vi "Main.vi"() -> ()   [LabVIEW 2016]
doc: "This template is for the Queued Message Handler design pattern.\n\nThe Event Handling Loop generates messages based on user interface actions.\n\nThe Message Handling Loop processes messages generated by the Event Handling Loop, or by other messages. The messages are string values, so new messages can be added easily to the Message Cases case structure in the Message Handling Loop. Each message cluster can also provide an optional value for Message Data, which is a variant that can be converted to whatever message-specific data is required."
uses:
  <vilib>/Utility/error.llb/Error Cluster From Error Code.vi
  <vilib>/ErrorRing/Error Ring.xnode
  3.SubVI/Message Queue/Message Queue.lvlib
panel:
  in  "Tab Control":enum32{"Page 1", "Page 2"}(tab)
  out "Display":string
  in  "Cancel Button":bool
  in  "原點復歸1":bool
  in  "生產結束":bool
  in  "Recipe":bool
  in  "Setting":bool
  in  "System":bool
  in  "停止":bool
  in  "啟動":bool
  out "X":dbl
  out "Y":dbl
  out "ON/OFF":bool
  in  "Pause":bool
  out "Speed":dbl
  in  "入料":bool
  in  "入料 2":bool
  out "Speed 2":dbl
  out "Y 2":dbl
  out "X 2":dbl
  out "ON/OFF 2":bool
  out "Display  2":string
  in  "原點復歸2":bool
  in  "Pause 2":bool
  in  "Cancel Button 2":bool
  in  "復歸":bool
  in  "SVON":bool
  in  "U":bool
  in  "D":bool
  in  "L":bool
  in  "R":bool
  in  "Step Ring 2":u16(ring) items=["0.001 mm", "0.01 mm", "0.1 mm", "1 mm"]
  in  "Jog_Speed":i32=10000
  # "工具列"
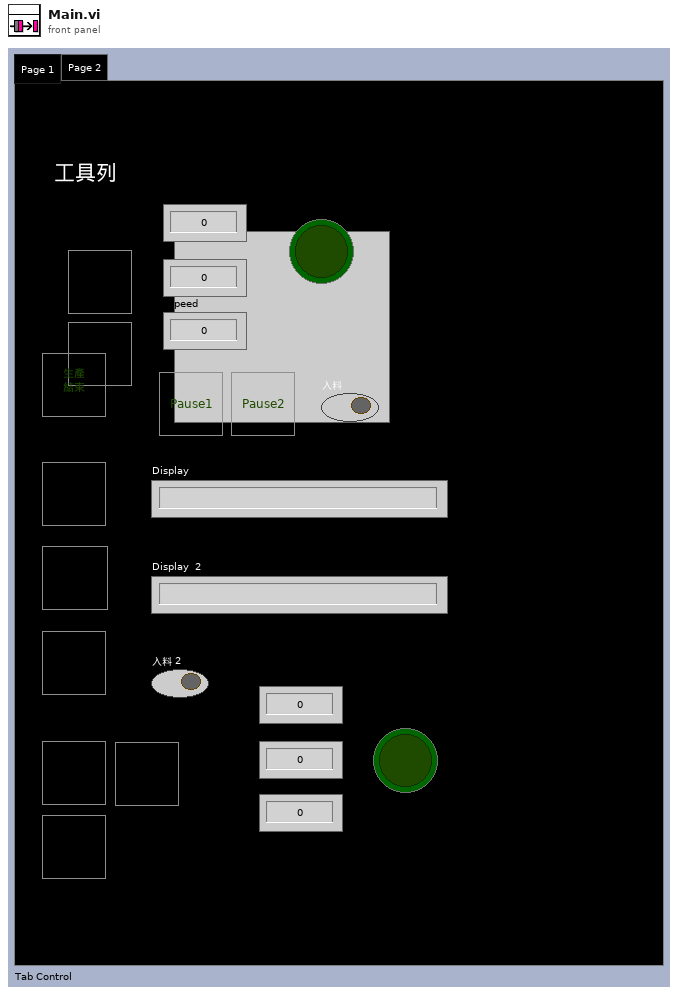
[diagram p1: front panel]
types:
  T1 = enum16{"Open", "Enqueue", "InsertQueue", "Release Queue", "Close"}
  T2 = enum16{"Open", "Move", "Check done", "E.Stop", "Get posion", "Home", "Serv ON/OFF", "Reset Error", "Set Param", "Close"}
  T3 = cluster{"X":dbl, "Y":dbl, "Speed":dbl, "Message":string}[]
  T4 = cluster{"X":dbl, "Y":dbl, "Speed":dbl, "Message":string}
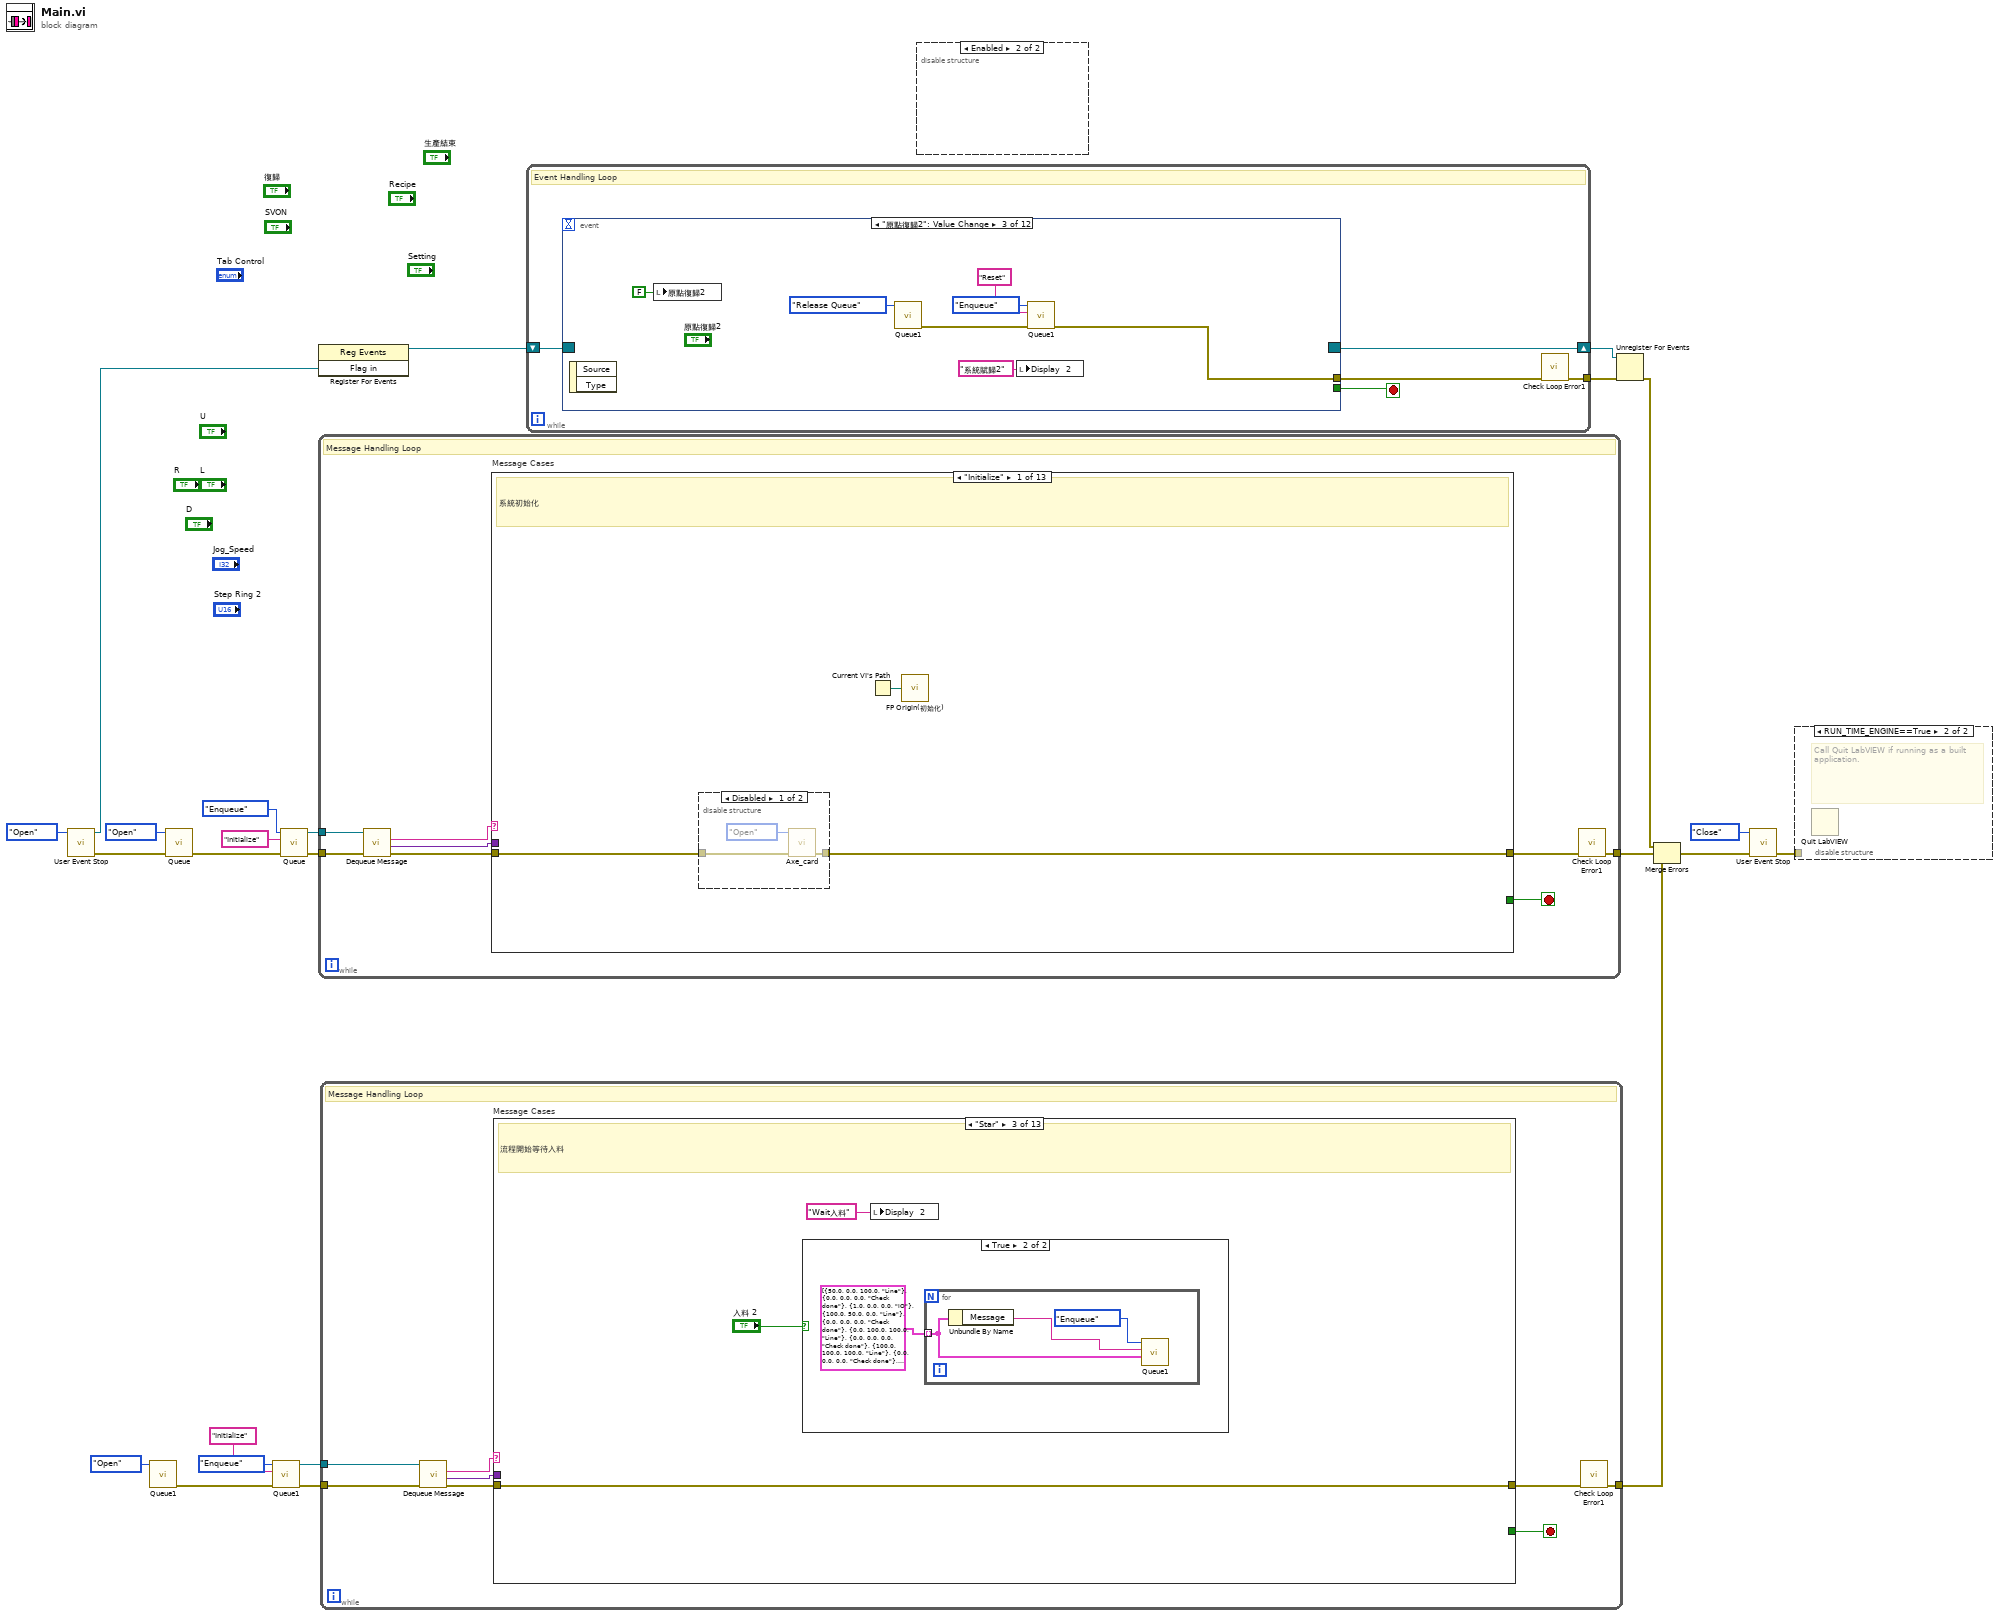
[diagram p0: block diagram]
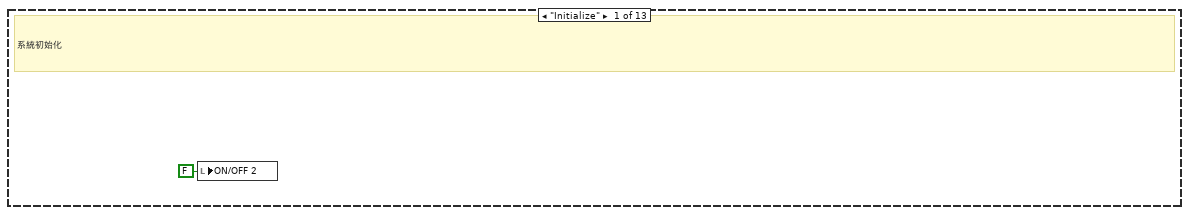
[diagram p2: hidden frame]
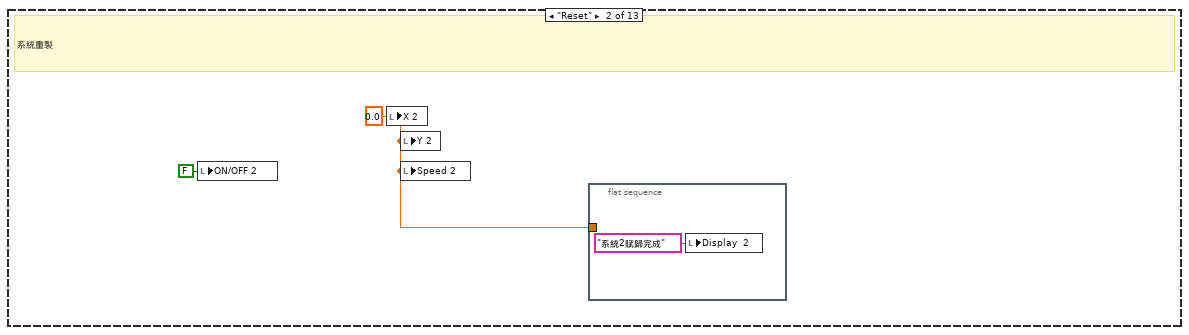
[diagram p3: hidden frame]
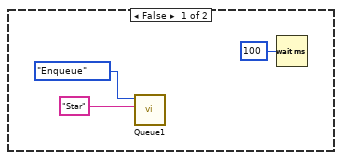
[diagram p4: hidden frame]
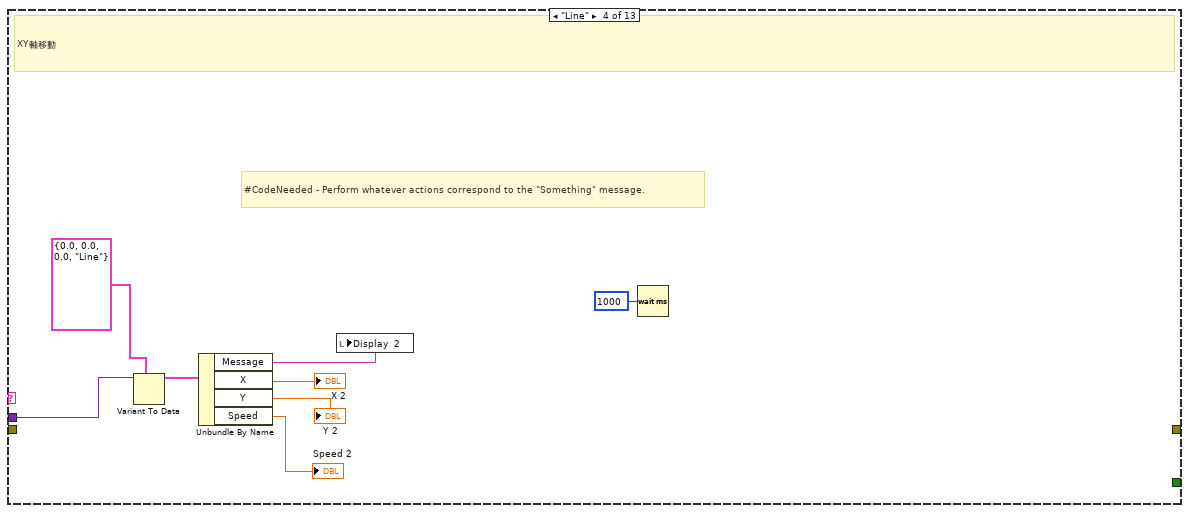
[diagram p5: hidden frame]
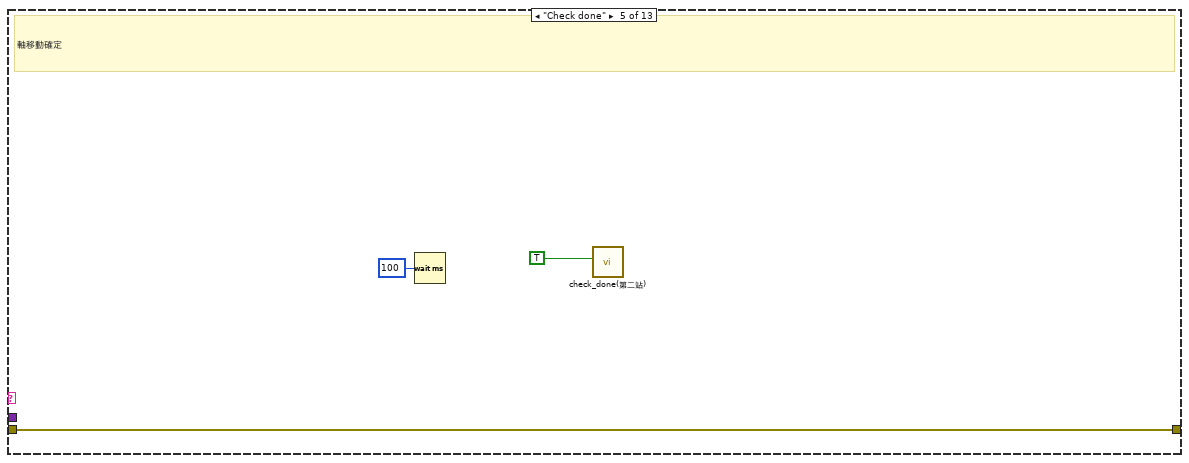
[diagram p6: hidden frame]
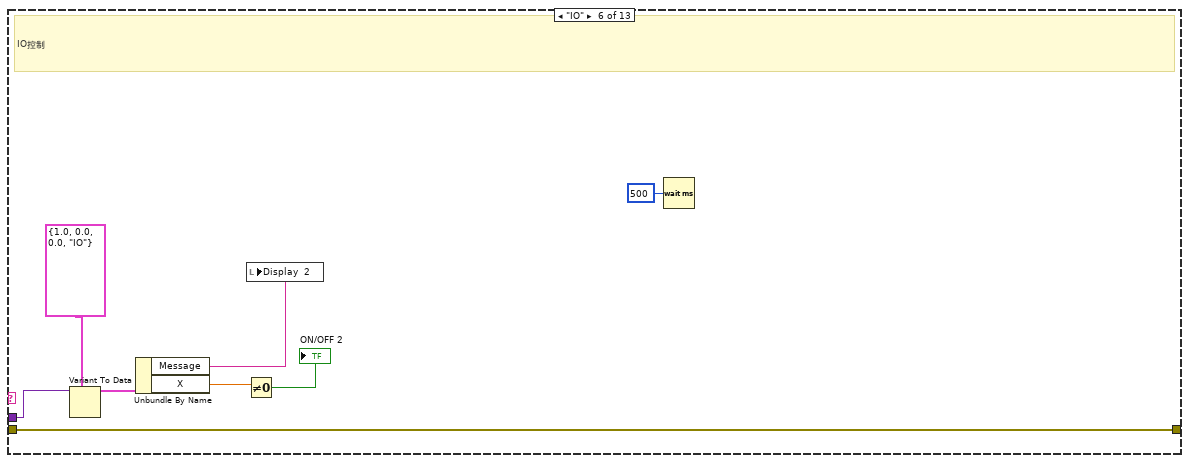
[diagram p7: hidden frame]
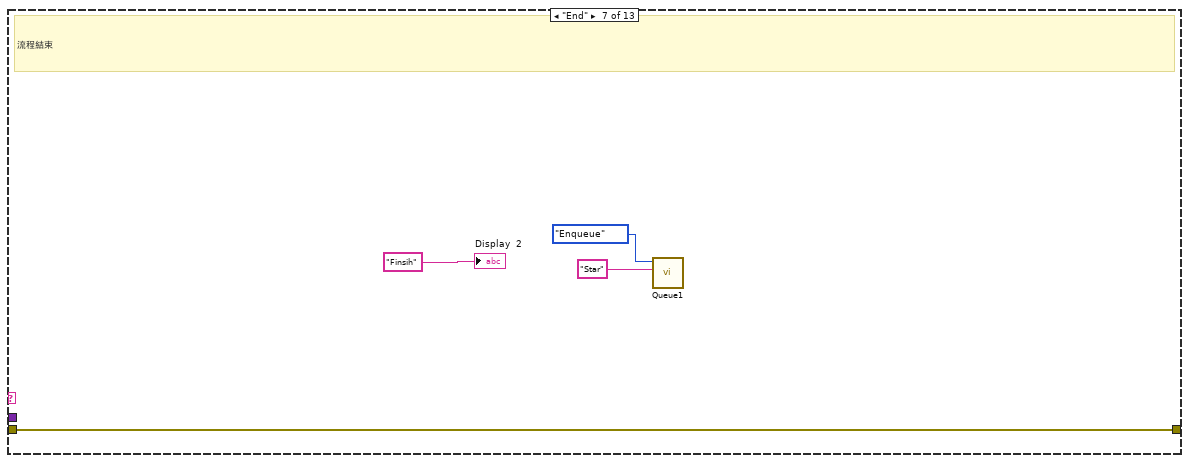
[diagram p8: hidden frame]
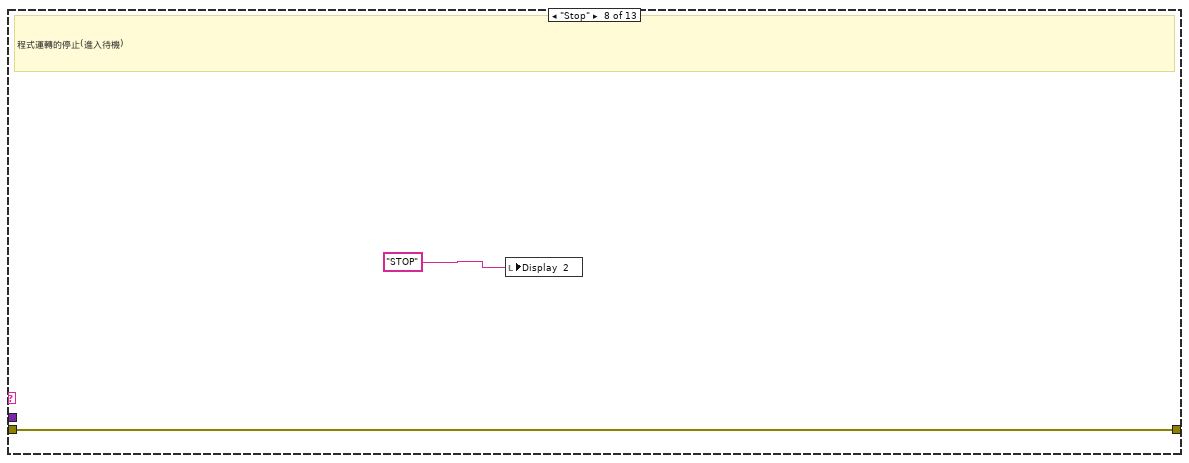
[diagram p9: hidden frame]
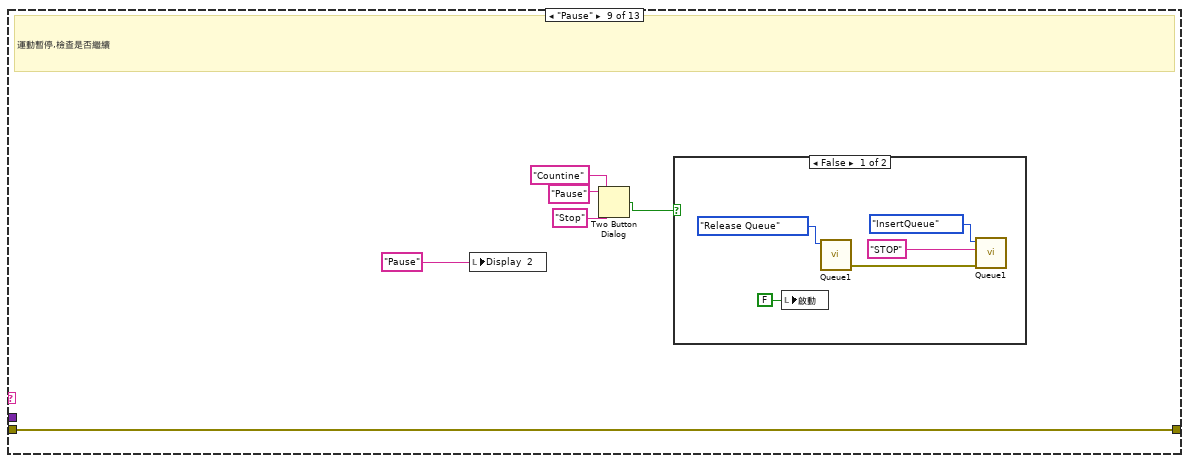
[diagram p10: hidden frame]
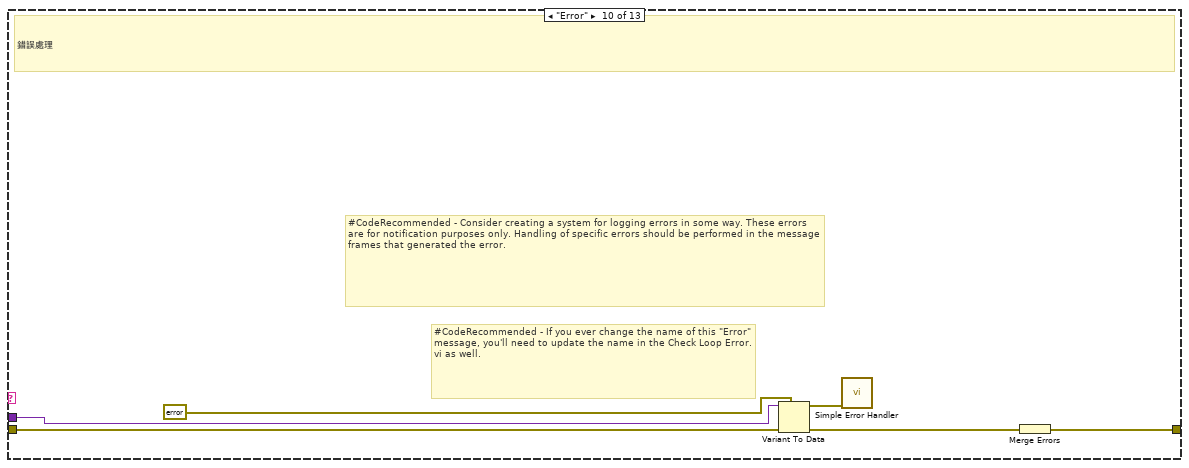
[diagram p12: hidden frame]
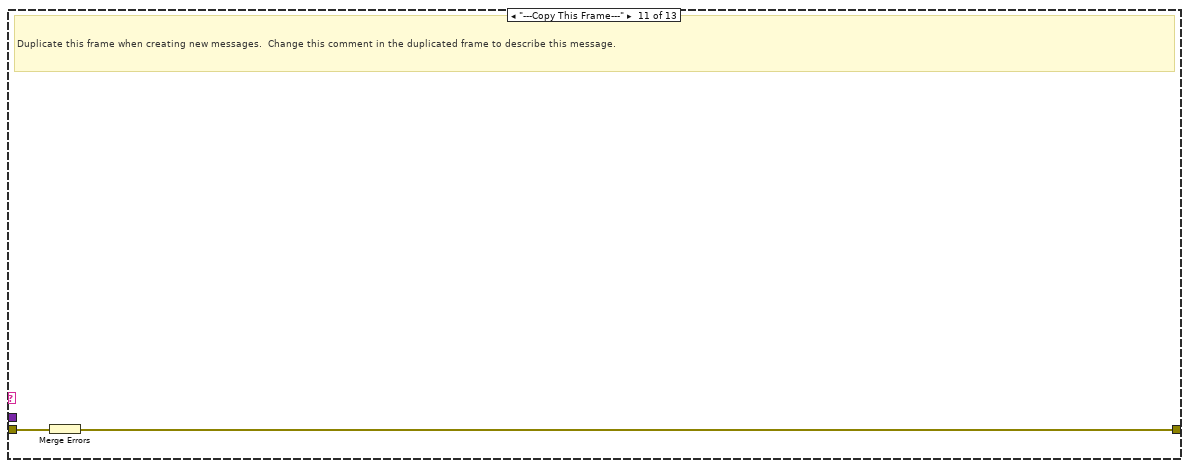
[diagram p13: hidden frame]
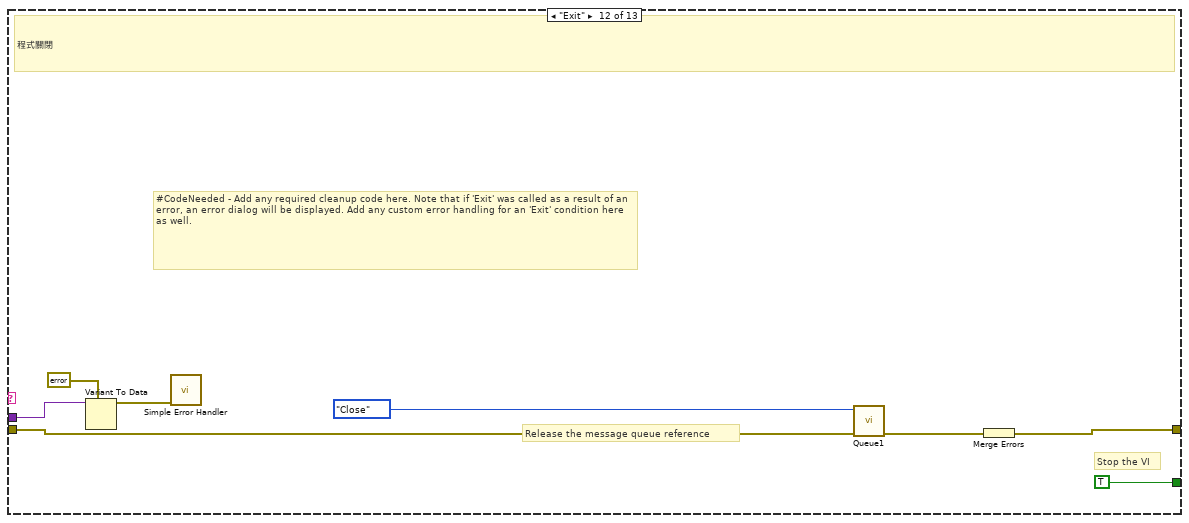
[diagram p14: hidden frame]
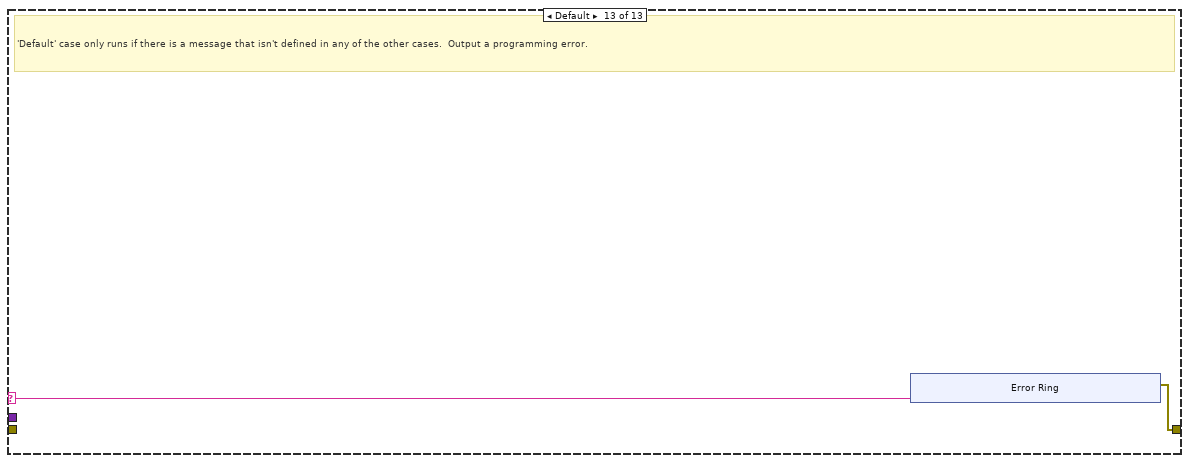
[diagram p15: hidden frame]
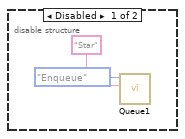
[diagram p16: hidden frame]
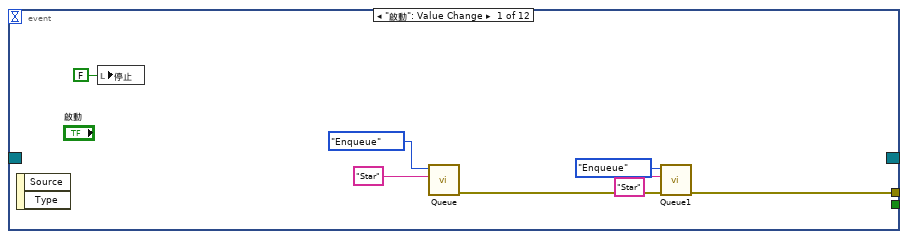
[diagram p18: hidden frame]
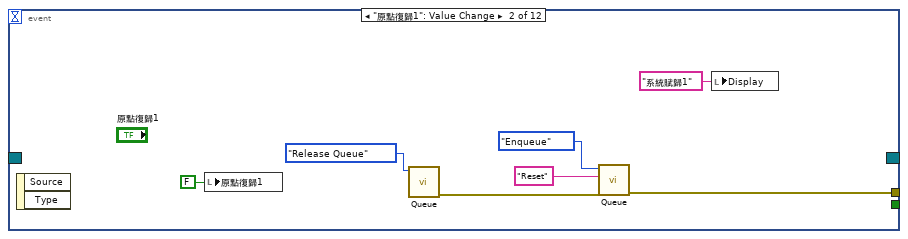
[diagram p19: hidden frame]
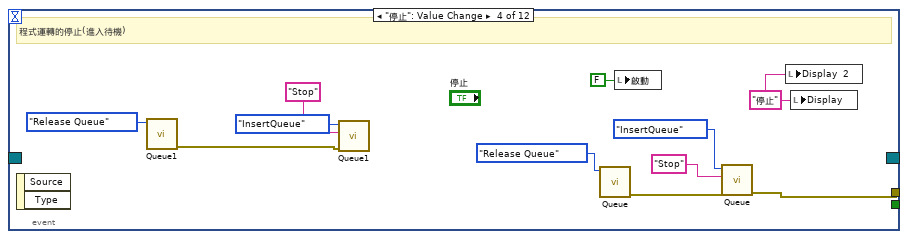
[diagram p20: hidden frame]
diagram:
  n1 = call "User Event Stop.vi"("Function"=enum16{"Open", "Event Write", "Close"}."Open") -> ("error out"=w13:errorcluster, "Flag in"=w14:refnum<user-event>)  [unwired: 9 in]
  n2 = call "Queue1.vi"("Function"=T1."Open") -> ("error out"=w6:errorcluster)  [unwired: 8 in, 2 out]
  n3 = call "Queue.vi"("error in"=w13, "Function"=T1."Open") -> ("error out"=w18:errorcluster)  [unwired: 7 in, 2 out]
  n4 = call "Queue1.vi"("error in"=w6, "Message"="Initialize", "Function"=T1."Enqueue") -> ("error out"=w1:errorcluster, "queue out"=w2:refnum<queue>)  [unwired: 6 in, 1 out]
  n5 = call "Queue.vi"("error in"=w18, "Message"="Initialize", "Function"=T1."Enqueue") -> ("error out"=w15:errorcluster, "queue out"=w16:refnum<queue>)  [unwired: 6 in, 1 out]
  n6 = register-events(w14) -> (reference out=w8:refnum<event-registration>)  [unwired: 2 in, 1 out]
  n7 = while {
    tunnel: w16 -> [w27]
    tunnel: w15 -> [w31]
    tunnel: [w25] -> w24
    stop <- w32 stop-if-true
    # "Message Handling Loop"
    n8 = call "Dequeue Message.vi"("error in (no error)"=w31, "Message Queue"=w27) -> ("error out"=w30:errorcluster, "Message Data"=w28:variant, "Message"=w29:string)  [unwired: 6 in, 1 out]
    n9 = case "Message Cases" shown="\"Initialize\"" w29 {
      selector: w29 -> [_ _ _ w60 _ _ _ _ _ _ _ _ w125]
      tunnel: w30 -> [w34 _ w43 _ w70 w78 w80 w85 w87 w111 w113 w118 _]
      tunnel: [w33 _ w42 _ w70 w78 w79 w85 w86 w106 w112 w123 w126] -> w26
      tunnel: [_ _ _ _ _ _ _ _ _ _ _ TRUE _] -> w32
      tunnel: w28 -> [_ _ _ w59 _ w77 _ _ _ w110 _ w120 _]
      frame "Initialize" {
        # "系統初始化"
        n10 = disable-structure shown="Disabled" {
          disable-tunnel: w34 -> [w38 _]
          disable-tunnel: [w37 _] -> w33
          frame Disabled {
            n11 = call "Axe_card.vi"("error in (no error)"=w38, "Function"=T2."Open") -> ("error out"=w37:errorcluster)  [unwired: 6 in, 3 out]
          }
          frame Enabled {
          }
        }
        n12 = Current VI's Path() -> (path=w35:path)
        n13 = call "FP Origin(初始化).vi"("vi path"=w35) -> ()  [unwired: 1 out]
      }
      frame "Reset" {
        w40 = 0.0 ("X")
        w39 = FALSE ("ON/OFF")
        # "系統重製"
        n14 = local write "停止"(w39) -> ()
        n15 = local write "啟動"(w39) -> ()
        n16 = local write "ON/OFF"(w39) -> ()
        n17 = local write "X"(w40) -> ()
        n18 = local write "Y"(w40) -> ()
        n19 = local write "Speed"(w40) -> ()
        n20 = flat-sequence {
          tunnel: w40 -> [_]
          frame #0 {
            n21 = local write "Display"("系統1賦歸完成" ("Display")) -> ()
          }
        }
      }
      frame "Star" {
        # "流程開始等待入料"
        n22 = local write "Display"("Wait入料" ("Display")) -> ()
        n23 = case shown="True" "入料" {
          tunnel: w43 -> [w47 w51]
          tunnel: [w46 w52] -> w42
          frame False {
            n24 = call "Queue.vi"("error in"=w47, "Message"="Star", "Function"=T1."Enqueue") -> ("error out"=w46:errorcluster)  [unwired: 6 in, 2 out]
            n25 = Wait (ms)(milliseconds to wait=u32 100) -> ()  [unwired: 1 out]
          }
          frame True {
            n26 = for {
              tunnel: T3 [{"X"=2.0, "Y"=0.0, "Speed"=100.0, "Message"="Line"}, {"X"=0.0, "Y"=0.0, "Speed"=0.0, "Message"="Check done"}, {"X"=1.0, "Y"=0.0, "Speed"=0.0, "Message"="IO"}, {"X"=100.0, "Y"=0.0, "Speed"=0.0, "Message"="Line"}, {"X"=0.0, "Y"=0.0, "Speed"=0.0, "Message"="Check done"}, {"X"=0.0, "Y"=100.0, "Speed"=100.0, "Message"="Line"}, {"X"=0.0, "Y"=0.0, "Speed"=0.0, "Message"="Check done"}, {"X"=100.0, "Y"=100.0, "Speed"=100.0, "Message"="Line"}, {"X"=0.0, "Y"=0.0, "Speed"=0.0, "Message"="Check done"}, {"X"=0.0, "Y"=100.0, "Speed"=100.0, "Message"="Line"}, {"X"=0.0, "Y"=0.0, "Speed"=0.0, "Message"="Check done"}, {"X"=0.0, "Y"=0.0, "Speed"=0.0, "Message"="IO"}, {"X"=20.0, "Y"=20.0, "Speed"=100.0, "Message"="Line"}, {"X"=0.0, "Y"=0.0, "Speed"=0.0, "Message"="Check done"}, {"X"=1.0, "Y"=0.0, "Speed"=0.0, "Message"="IO"}, {"X"=20.0, "Y"=20.0, "Speed"=100.0, "Message"="Line"}, {"X"=0.0, "Y"=0.0, "Speed"=0.0, "Message"="Check done"}, {"X"=20.0, "Y"=80.0, "Speed"=100.0, "Message"="Line"}, {"X"=0.0, "Y"=0.0, "Speed"=0.0, "Message"="Check done"}, {"X"=0.0, "Y"=0.0, "Speed"=0.0, "Message"="IO"}, {"X"=0.0, "Y"=0.0, "Speed"=0.0, "Message"="Line"}, {"X"=0.0, "Y"=0.0, "Speed"=0.0, "Message"="End"}] -> [w57] mode=indexing
              shift-right: [w54] -> w52
              shift-left: w51 -> [w55]
              n27 = Unbundle By Name(w57) -> ("Message"=w56:string)
              n28 = call "Queue.vi"("error in"=w55, "Message Data"=w57, "Message"=w56, "Function"=T1."Enqueue") -> ("error out"=w54:errorcluster)  [unwired: 5 in, 2 out]
            }
          }
        }
      }
      frame "Line" {
        # "#CodeNeeded - Perform whatever actions correspond to the \"Something\" message."
        # "XY軸移動"
        n29 = call "Line_FGV.vi"("Message Data"=w59, "Message"=w60) -> ()  [unwired: 7 in, 3 out]
        n30 = Variant To Data(type=T4 {"X"=0.0, "Y"=0.0, "Speed"=0.0, "Message"="Line"}, Variant=w59) -> (data=w66:T4)  [unwired: 1 in, 1 out]
        n31 = Unbundle By Name(w66) -> ("Message"=w62:string, "X"=→"X":dbl, "Y"=→"Y":dbl, "Speed"=→"Speed":dbl)
        n32 = local write "Display"(w62) -> ()
        n33 = Wait (ms)(milliseconds to wait=u32 1000) -> ()  [unwired: 1 out]
      }
      frame "Check done" {
        # "軸移動確定"
        n34 = Wait (ms)(milliseconds to wait=u32 100) -> ()  [unwired: 1 out]
        n35 = call "check_done.vi"("Boolean"=TRUE) -> ()  [unwired: 10 in, 1 out]
      }
      frame "IO" {
        # "IO控制"
        n36 = Variant To Data(type=T4 {"X"=1.0, "Y"=0.0, "Speed"=0.0, "Message"="IO"}, Variant=w77) -> (data=w75:T4)  [unwired: 1 in, 1 out]
        n37 = Unbundle By Name(w75) -> ("Message"=w71:string, "X"=w74:dbl)
        n38 = Not Equal To 0?(x=w74) -> (x != 0?=→"ON/OFF":bool)
        n39 = local write "Display"(w71) -> ()
        n40 = Wait (ms)(milliseconds to wait=u32 500) -> ()  [unwired: 1 out]
      }
      frame "End" {
        # "流程結束"
        n41 = call "Queue.vi"("error in"=w80, "Message"="Star", "Function"=T1."Enqueue") -> ("error out"=w79:errorcluster)  [unwired: 6 in, 2 out]
        "Display" <- "Finsih" ("Display <Replace Me>")
      }
      frame "Stop" {
        # "程式運轉的停止(進入待機)"
        n42 = local write "Display"("STOP" ("Display <Replace Me>")) -> ()
      }
      frame "Pause" {
        # "運動暫停,檢查是否繼續"
        n43 = local write "Display"("Pause" ("Display <Replace Me>")) -> ()
        n44 = Two Button Dialog(message="Pause", 1:"Stop" ("F button name (\"Cancel\")"), 2:"Countine" ("T button name (\"OK\")")) -> (T button?=w89:bool)
        n45 = case shown="True" w89 {
          tunnel: w87 -> [w94 w101]
          tunnel: [w93 w102] -> w86
          frame False {
            n46 = local write "啟動"(FALSE ("啟動")) -> ()
            n47 = call "Queue.vi"("error in"=w94, "Function"=T1."Release Queue") -> ("error out"=w99:errorcluster)  [unwired: 7 in, 2 out]
            n48 = call "Queue.vi"("error in"=w99, "Message"="STOP", "Function"=T1."InsertQueue") -> ("error out"=w93:errorcluster)  [unwired: 6 in, 2 out]
          }
          frame True {
            # "Line位置再被執行一次"
            n49 = call "Line_FGV.vi"("error in (no error)"=w101) -> ("error out"=w100:errorcluster, "Message Data 2"=w103:variant, "Message 2"=w104:string)  [unwired: 8 in]
            n50 = call "Queue.vi"("error in"=w100, "Message Data"=w103, "Message"=w104, "Function"=T1."InsertQueue") -> ("error out"=w102:errorcluster)  [unwired: 5 in, 2 out]
          }
        }
      }
      frame "Error" {
        # "#CodeRecommended - If you ever change the name of this \"Error\" message, you'll need to update the name in the Check Loop Error.vi as well."
        # "#CodeRecommended - Consider creating a system for logging errors in some way. These errors are for notification purposes only. Handling of specific errors should be performed in the message frames that generated the error."
        # "錯誤處理"
        n51 = Variant To Data(error in=w111, type=errorcluster {"status"=FALSE, "code"=0, "source"=""} ("error constant"), Variant=w110) -> (data=w108:errorcluster, error out=w107:errorcluster)
        n52 = call <vilib>:"Simple Error Handler.vi"("error in (no error)"=w108) -> ()  [unwired: 4 in, 5 out]
        n53 = Merge Errors(w107) -> (w106:errorcluster)
      }
      frame "---Copy This Frame---" {
        # "Duplicate this frame when creating new messages.  Change this comment in the duplicated frame to describe this message."
        n54 = Merge Errors(w113) -> (w112:errorcluster)
      }
      frame "Exit" {
        # "Stop the VI"
        # "Release the message queue reference"
        # "#CodeNeeded - Add any required cleanup code here. Note that if 'Exit' was called as a result of an error, an error dialog will be displayed. Add any custom error handling for an 'Exit' condition here as well."
        # "程式關閉"
        n55 = Variant To Data(type=errorcluster {"status"=FALSE, "code"=0, "source"=""} ("error constant"), Variant=w120) -> (data=w121:errorcluster)  [unwired: 1 in, 1 out]
        n56 = call <vilib>:"Simple Error Handler.vi"("error in (no error)"=w121) -> ()  [unwired: 4 in, 5 out]
        n57 = call "Queue.vi"("error in"=w118, "Function"=T1."Close") -> ("error out"=w117:errorcluster)  [unwired: 7 in, 2 out]
        n58 = call "User Event Stop.vi"("event data"=TRUE, "Function"=enum16{"Open", "Event Write", "Close"}."Event Write") -> ("error out"=w115:errorcluster)  [unwired: 8 in, 1 out]
        n59 = Merge Errors(w115, w117) -> (w123:errorcluster)
      }
      frame Default {
        # "'Default' case only runs if there is a message that isn't defined in any of the other cases.  Output a programming error."
        n60 = xnode "Error Ring"("parameter 0"=w125) -> ("error out"=w126:errorcluster)
      }
    }
    n61 = call "Check Loop Error1.vi"("dup error in"=w26) -> ("Error Out"=w25:errorcluster)  [unwired: 10 in]
  }
  n62 = while {
    tunnel: w2 -> [w136]
    tunnel: w1 -> [w140]
    tunnel: [w134] -> w3
    stop <- w141 stop-if-true
    # "Message Handling Loop"
    n63 = call "Dequeue Message.vi"("error in (no error)"=w140, "Message Queue"=w136) -> ("error out"=w139:errorcluster, "Message Data"=w137:variant, "Message"=w138:string)  [unwired: 6 in, 1 out]
    n64 = case "Message Cases" shown="\"Star\"" w138 {
      selector: w138 -> [_ _ _ _ _ _ _ _ _ _ _ _ w208]
      tunnel: w139 -> [_ _ w148 _ w166 w174 w178 w180 w186 w197 w199 w201 _]
      tunnel: [_ _ w148 _ w166 w174 w178 w180 w186 w192 w198 w206 w209] -> w135
      tunnel: [_ _ _ _ _ _ _ _ _ _ _ TRUE _] -> w141
      tunnel: w137 -> [_ _ _ w163 _ w173 _ _ _ w196 _ w203 _]
      frame "Initialize" {
        # "系統初始化"
        n65 = local write "ON/OFF 2"(FALSE ("ON/OFF")) -> ()
      }
      frame "Reset" {
        w143 = 0.0 ("X")
        # "系統重製"
        n66 = local write "ON/OFF 2"(FALSE ("ON/OFF")) -> ()
        n67 = local write "X 2"(w143) -> ()
        n68 = local write "Y 2"(w143) -> ()
        n69 = local write "Speed 2"(w143) -> ()
        n70 = flat-sequence {
          tunnel: w143 -> [_]
          frame #0 {
            n71 = local write "Display  2"("系統2賦歸完成" ("Display")) -> ()
          }
        }
      }
      frame "Star" {
        # "流程開始等待入料"
        n72 = case shown="True" "入料 2" {
          frame False {
            n73 = call "Queue1.vi"("Message"="Star", "Function"=T1."Enqueue") -> ()  [unwired: 7 in, 3 out]
            n74 = Wait (ms)(milliseconds to wait=u32 100) -> ()  [unwired: 1 out]
          }
          frame True {
            n75 = for {
              tunnel: T3 [{"X"=50.0, "Y"=0.0, "Speed"=100.0, "Message"="Line"}, {"X"=0.0, "Y"=0.0, "Speed"=0.0, "Message"="Check done"}, {"X"=1.0, "Y"=0.0, "Speed"=0.0, "Message"="IO"}, {"X"=100.0, "Y"=50.0, "Speed"=0.0, "Message"="Line"}, {"X"=0.0, "Y"=0.0, "Speed"=0.0, "Message"="Check done"}, {"X"=0.0, "Y"=100.0, "Speed"=100.0, "Message"="Line"}, {"X"=0.0, "Y"=0.0, "Speed"=0.0, "Message"="Check done"}, {"X"=100.0, "Y"=100.0, "Speed"=100.0, "Message"="Line"}, {"X"=0.0, "Y"=0.0, "Speed"=0.0, "Message"="Check done"}, {"X"=0.0, "Y"=100.0, "Speed"=100.0, "Message"="Line"}, {"X"=0.0, "Y"=0.0, "Speed"=0.0, "Message"="Check done"}, {"X"=0.0, "Y"=0.0, "Speed"=0.0, "Message"="IO"}, {"X"=20.0, "Y"=20.0, "Speed"=100.0, "Message"="Line"}, {"X"=0.0, "Y"=0.0, "Speed"=0.0, "Message"="Check done"}, {"X"=1.0, "Y"=0.0, "Speed"=0.0, "Message"="IO"}, {"X"=20.0, "Y"=20.0, "Speed"=100.0, "Message"="Line"}, {"X"=0.0, "Y"=0.0, "Speed"=0.0, "Message"="Check done"}, {"X"=20.0, "Y"=80.0, "Speed"=100.0, "Message"="Line"}, {"X"=0.0, "Y"=0.0, "Speed"=0.0, "Message"="Check done"}, {"X"=0.0, "Y"=0.0, "Speed"=0.0, "Message"="End"}] -> [w154] mode=indexing
              n76 = Unbundle By Name(w154) -> ("Message"=w153:string)
              n77 = call "Queue1.vi"("Message Data"=w154, "Message"=w153, "Function"=T1."Enqueue") -> ()  [unwired: 6 in, 3 out]
            }
          }
        }
        n78 = local write "Display  2"("Wait入料" ("Display")) -> ()
      }
      frame "Line" {
        # "#CodeNeeded - Perform whatever actions correspond to the \"Something\" message."
        # "XY軸移動"
        n79 = Variant To Data(type=T4 {"X"=0.0, "Y"=0.0, "Speed"=0.0, "Message"="Line"}, Variant=w163) -> (data=w161:T4)  [unwired: 1 in, 1 out]
        n80 = Unbundle By Name(w161) -> ("Message"=w157:string, "X"=→"X 2":dbl, "Y"=→"Y 2":dbl, "Speed"=→"Speed 2":dbl)
        n81 = local write "Display  2"(w157) -> ()
        n82 = Wait (ms)(milliseconds to wait=u32 1000) -> ()  [unwired: 1 out]
      }
      frame "Check done" {
        # "軸移動確定"
        n83 = Wait (ms)(milliseconds to wait=u32 100) -> ()  [unwired: 1 out]
        n84 = call "check_done(第二站).vi"("Boolean"=TRUE) -> ()  [unwired: 10 in, 1 out]
      }
      frame "IO" {
        # "IO控制"
        n85 = Variant To Data(type=T4 {"X"=1.0, "Y"=0.0, "Speed"=0.0, "Message"="IO"}, Variant=w173) -> (data=w171:T4)  [unwired: 1 in, 1 out]
        n86 = Unbundle By Name(w171) -> ("Message"=w167:string, "X"=w170:dbl)
        n87 = Not Equal To 0?(x=w170) -> (x != 0?=→"ON/OFF 2":bool)
        n88 = local write "Display  2"(w167) -> ()
        n89 = Wait (ms)(milliseconds to wait=u32 500) -> ()  [unwired: 1 out]
      }
      frame "End" {
        # "流程結束"
        n90 = call "Queue1.vi"("Message"="Star", "Function"=T1."Enqueue") -> ()  [unwired: 7 in, 3 out]
        "Display  2" <- "Finsih" ("Display <Replace Me>")
      }
      frame "Stop" {
        # "程式運轉的停止(進入待機)"
        n91 = local write "Display  2"("STOP" ("Display <Replace Me>")) -> ()
      }
      frame "Pause" {
        # "運動暫停,檢查是否繼續"
        n92 = local write "Display  2"("Pause" ("Display <Replace Me>")) -> ()
        n93 = Two Button Dialog(message="Pause", 1:"Stop" ("F button name (\"Cancel\")"), 2:"Countine" ("T button name (\"OK\")")) -> (T button?=w182:bool)
        n94 = case shown="False" w182 {
          frame False {
            n95 = local write "啟動"(FALSE ("啟動")) -> ()
            n96 = call "Queue1.vi"("Function"=T1."Release Queue") -> ("error out"=w191:errorcluster)  [unwired: 8 in, 2 out]
            n97 = call "Queue1.vi"("error in"=w191, "Message"="STOP", "Function"=T1."InsertQueue") -> ()  [unwired: 6 in, 3 out]
          }
          frame True {
          }
        }
      }
      frame "Error" {
        # "#CodeRecommended - If you ever change the name of this \"Error\" message, you'll need to update the name in the Check Loop Error.vi as well."
        # "#CodeRecommended - Consider creating a system for logging errors in some way. These errors are for notification purposes only. Handling of specific errors should be performed in the message frames that generated the error."
        # "錯誤處理"
        n98 = Variant To Data(error in=w197, type=errorcluster {"status"=FALSE, "code"=0, "source"=""} ("error constant"), Variant=w196) -> (data=w194:errorcluster, error out=w193:errorcluster)
        n99 = call <vilib>:"Simple Error Handler.vi"("error in (no error)"=w194) -> ()  [unwired: 4 in, 5 out]
        n100 = Merge Errors(w193) -> (w192:errorcluster)
      }
      frame "---Copy This Frame---" {
        # "Duplicate this frame when creating new messages.  Change this comment in the duplicated frame to describe this message."
        n101 = Merge Errors(w199) -> (w198:errorcluster)
      }
      frame "Exit" {
        # "Stop the VI"
        # "Release the message queue reference"
        # "#CodeNeeded - Add any required cleanup code here. Note that if 'Exit' was called as a result of an error, an error dialog will be displayed. Add any custom error handling for an 'Exit' condition here as well."
        # "程式關閉"
        n102 = Variant To Data(type=errorcluster {"status"=FALSE, "code"=0, "source"=""} ("error constant"), Variant=w203) -> (data=w204:errorcluster)  [unwired: 1 in, 1 out]
        n103 = call <vilib>:"Simple Error Handler.vi"("error in (no error)"=w204) -> ()  [unwired: 4 in, 5 out]
        n104 = call "Queue1.vi"("error in"=w201, "Function"=T1."Close") -> ("error out"=w200:errorcluster)  [unwired: 7 in, 2 out]
        n105 = Merge Errors(w200) -> (w206:errorcluster)
      }
      frame Default {
        # "'Default' case only runs if there is a message that isn't defined in any of the other cases.  Output a programming error."
        n106 = xnode "Error Ring"("parameter 0"=w208) -> ("error out"=w209:errorcluster)
      }
    }
    n107 = call "Check Loop Error1.vi"("dup error in"=w135) -> ("Error Out"=w134:errorcluster)  [unwired: 10 in]
  }
  n108 = while {
    shift-right: [w221] -> w22
    shift-left: w8 -> [w217]
    tunnel: [w218] -> w21
    stop <- w220 stop-if-true
    # "Event Handling Loop"
    n109 = event shown="[2] \"原點復歸2\": Value Change" {
      selector: w217 -> [_ _ _ _ _ _ _ _ _ _ _ _]
      dyn-events: [_ _ _ _ _ _ _ _ _ _ _ _] -> w221
      timeout: _ -> [_ _ _ _ _ _ _ _ _ _ _ _]
      tunnel: [_ _ _ _ _ _ _ _ _ _ _ TRUE ("Discard?")] -> w220
      tunnel: [w222 w232 w239 w248 _ _ _ _ _ _ _ _] -> w219
      event "啟動": Value Change {
        n110 = event-data() -> ()  [unwired: 1 in, 2 out]
        n111 = local write "停止"(FALSE ("停止")) -> ()
        n112 = call "Queue.vi"("Message"="Star", "Function"=T1."Enqueue") -> ("error out"=w223:errorcluster)  [unwired: 7 in, 2 out]
        n113 = call "Queue1.vi"("error in"=w223, "Message"="Star", "Function"=T1."Enqueue") -> ("error out"=w222:errorcluster)  [unwired: 6 in, 2 out]
      }
      event "原點復歸1": Value Change {
        n114 = event-data() -> ()  [unwired: 1 in, 2 out]
        n115 = local write "原點復歸1"(FALSE ("原點復歸1")) -> ()
        n116 = call "Queue.vi"("Function"=T1."Release Queue") -> ("error out"=w229:errorcluster)  [unwired: 8 in, 2 out]
        n117 = call "Queue.vi"("error in"=w229, "Message"="Reset", "Function"=T1."Enqueue") -> ("error out"=w232:errorcluster)  [unwired: 6 in, 2 out]
        n118 = local write "Display"("系統賦歸1" ("Display")) -> ()
      }
      event "原點復歸2": Value Change {
        n119 = event-data() -> ()  [unwired: 1 in, 2 out]
        n120 = local write "原點復歸2"(FALSE ("原點復歸2")) -> ()
        n121 = call "Queue1.vi"("Function"=T1."Release Queue") -> ("error out"=w236:errorcluster)  [unwired: 8 in, 2 out]
        n122 = local write "Display  2"("系統賦歸2" ("Display")) -> ()
        n123 = call "Queue1.vi"("error in"=w236, "Message"="Reset", "Function"=T1."Enqueue") -> ("error out"=w239:errorcluster)  [unwired: 6 in, 2 out]
      }
      event "停止": Value Change {
        w243 = "停止" ("Display")
        # "程式運轉的停止(進入待機)"
        n124 = event-data() -> ()  [unwired: 1 in, 2 out]
        n125 = call "Queue1.vi"("Function"=T1."Release Queue") -> ("error out"=w244:errorcluster)  [unwired: 8 in, 2 out]
        n126 = call "Queue1.vi"("error in"=w244, "Message"="Stop", "Function"=T1."InsertQueue") -> ()  [unwired: 6 in, 3 out]
        n127 = call "Queue.vi"("Function"=T1."Release Queue") -> ("error out"=w249:errorcluster)  [unwired: 8 in, 2 out]
        n128 = local write "啟動"(FALSE ("啟動")) -> ()
        n129 = call "Queue.vi"("error in"=w249, "Message"="Stop", "Function"=T1."InsertQueue") -> ("error out"=w248:errorcluster)  [unwired: 6 in, 2 out]
        n130 = local write "Display  2"(w243) -> ()
        n131 = local write "Display"(w243) -> ()
      }
      event "System": Value Change {
        n132 = event-data() -> ()  [unwired: 1 in, 2 out]
        n133 = local write "System"(FALSE ("System")) -> ()
        n134 = local write "Tab Control"(enum32{"Page 1", "Page 2"}."Page 2" ("Tab Control")) -> ()
      }
      event "Cancel Button 2": Value Change {
        n135 = event-data() -> ()  [unwired: 1 in, 2 out]
        n136 = local write "Cancel Button 2"(FALSE ("Cancel Button 2")) -> ()
        n137 = local write "Tab Control"(enum32{"Page 1", "Page 2"}."Page 1" ("Tab Control")) -> ()
      }
      event "Pause": Value Change {
        n138 = event-data() -> ()  [unwired: 1 in, 2 out]
        n139 = call "Queue.vi"("Message"="Pause", "Function"=T1."InsertQueue") -> ()  [unwired: 7 in, 3 out]
        n140 = local write "Pause"(FALSE ("Pause")) -> ()
      }
      event "Pause 2": Value Change {
        n141 = event-data() -> ()  [unwired: 1 in, 2 out]
        n142 = call "Queue1.vi"("Message"="Pause", "Function"=T1."InsertQueue") -> ()  [unwired: 7 in, 3 out]
        n143 = local write "Pause 2"(FALSE ("Pause")) -> ()
      }
      event Panel Close? {
        n144 = event-data() -> ()  [unwired: 1 in, 1 out]
        n145 = Two Button Dialog(message="Cloase Program?", 1:"No" ("F button name (\"Cancel\")"), 2:"Yes" ("T button name (\"OK\")")) -> (T button?=w264:bool)
        n146 = case shown="True" w264 {
          frame False {
          }
          frame True {
            n147 = call "Queue.vi"("Message"="Exit", "Function"=T1."Enqueue") -> ("error out"=w269:errorcluster)  [unwired: 7 in, 2 out]
            n148 = call "Queue1.vi"("error in"=w269, "Message"="Exit", "Function"=T1."InsertQueue") -> ()  [unwired: 6 in, 3 out]
          }
        }
        n149 = event-data("Discard?"=TRUE) -> ()  [unwired: 1 in, 1 out]
      }
      event Application Instance Close {
        # "#CodeRecommended - When a project closes, all VIs within that project are aborted and leave memory. However, any code placed in this event frame is guaranteed to run to completion, so add any cleanup code that absolutely must happen here."
        n150 = event-data() -> ()  [unwired: 1 in, 1 out]
      }
      event "Cancel Button": Value Change {
        w275 = "Exit" ("Display")
        n151 = event-data() -> ()  [unwired: 1 in, 2 out]
        n152 = call "Queue.vi"("Message"="Exit", "Function"=T1."Enqueue") -> ("error out"=w274:errorcluster)  [unwired: 7 in, 2 out]
        n153 = call "Queue1.vi"("error in"=w274, "Message"="Exit", "Function"=T1."Enqueue") -> ()  [unwired: 6 in, 3 out]
        n154 = local write "Display  2"(w275) -> ()
        n155 = local write "Display"(w275) -> ()
      }
      event User Event {
        # "關閉介面控制"
        n156 = event-data() -> ()  [unwired: 1 in, 4 out]
      }
    }
    n157 = call "Check Loop Error1.vi"("dup error in"=w219) -> ("Error Out"=w218:errorcluster)  [unwired: 10 in]
  }
  n158 = disable-structure shown="Enabled" {
    frame Disabled {
      n159 = call "Queue1.vi"("Message"="Star", "Function"=T1."Enqueue") -> ()  [unwired: 7 in, 3 out]
    }
    frame Enabled {
    }
  }
  n160 = Unregister For Events(event registration refnum=w22, error in=w21) -> (error out=w23:errorcluster)
  n161 = Merge Errors(w23, w24, w3) -> (w10:errorcluster)
  n162 = call "User Event Stop.vi"("error in"=w10, "Function"=enum16{"Open", "Event Write", "Close"}."Close") -> ("error out"=w9:errorcluster)  [unwired: 8 in, 1 out]
  n163 = disable-structure shown="RUN_TIME_ENGINE==True" {
    disable-tunnel: w9 -> [_ _]
    frame condition #0 (active) {
    }
    frame condition #1 {
      # "Call Quit LabVIEW if running as a built application."
      n164 = Quit LabVIEW() -> ()  [unwired: 1 in]
    }
  }
